vi "题目2.vi"() -> ()   [LabVIEW 2017]
panel:
  out "数值 2":dbl
  out "数值":dbl
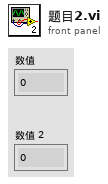
[diagram p1: front panel]
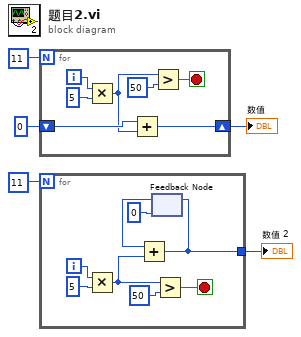
[diagram p0: block diagram]
diagram:
  n1 = for {
    N: 11 -> [_]
    shift-right: [w9] -> w3
    shift-left: 0 -> [w10]
    i -> [w11]
    stop <- w6 stop-if-true
    n2 = Multiply(x=w11, y=5) -> (x*y=w8:i32)
    n3 = Add(x=w10, y=w8) -> (x+y=w9:i32)
    n4 = Greater?(x=w8, y=50) -> (0:w6:bool)
  }
  "数值" <- w3
  n5 = for {
    N: 11 -> [_]
    tunnel: [w14] -> w2
    i -> [w20]
    stop <- w17 stop-if-true
    n6 = Multiply(x=w20, y=5) -> (x*y=w13:i32)
    n7 = feedback #1(0) -> (w15:i32)
    n8 = Add(x=w15, y=w13) -> (x+y=w14:i32)
    n9 = feedback-in #1(w14) -> ()
    n10 = Greater?(x=w13, y=50) -> (0:w17:bool)
  }
  "数值 2" <- w2
